vi "Initailize.vi"(8 "error in (no error)":errorcluster, 9 "zeromq.lvlib:ZeroMQ Context":refnum<class "zmq_context.lvclass">, 10 "Name":string, 11 "Channel Pub in":refnum<class "Channel Pub.lvclass">) -> (0 "error out":errorcluster, 3 "Channel Pub out":refnum<class "Channel Pub.lvclass">)   [LabVIEW 2018, in "Channel Pub.lvclass"]
uses:
  Channel Pub.lvclass
  <vilib>/addons/zeromq/zmq_context.lvclass
  Communication Channel/Communication Channel.lvclass
  Socket/Socket.lvclass
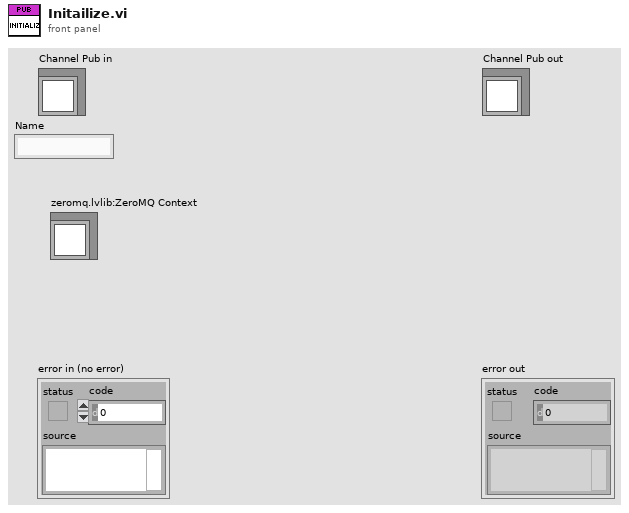
[diagram p1: front panel]
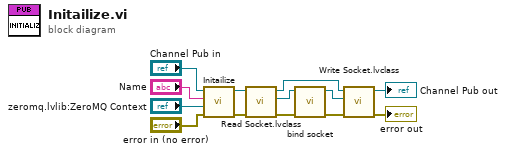
[diagram p0: block diagram]
diagram:
  n1 = call-parent "Initailize.vi"("error in (no error)"="error in (no error)", "zeromq.lvlib:ZeroMQ Context"="zeromq.lvlib:ZeroMQ Context", "Name"="Name", "Communication Channel in"="Channel Pub in") -> ("error out"=w5:errorcluster, "Communication Channel out"=w9:refnum<class "Channel Pub.lvclass">)  [unwired: 6 in]
  n2 = call-dynamic "Read Socket.lvclass.vi"("error in (no error)"=w5, "Communication Channel in"=w9) -> ("error out"=w4:errorcluster, "Socket.lvclass"=w8:refnum<class "Socket.lvclass">, "Communication Channel out"=w6:refnum<class "Channel Pub.lvclass">)  [unwired: 7 in]
  n3 = call "bind socket.vi"("error in (no error)"=w4, "Socket in"=w8) -> ("error out"=w3:errorcluster, "Socket out"=w7:refnum<class "Socket.lvclass">)  [unwired: 8 in]
  n4 = call-dynamic "Write Socket.lvclass.vi"("error in (no error)"=w3, "Socket2.lvclass"=w7, "Communication Channel in"=w6) -> ("error out"=→"error out":errorcluster, "Communication Channel out"=→"Channel Pub out":refnum<class "Channel Pub.lvclass">)  [unwired: 7 in]
